vi "Bulk Add Dialog.vi"(8 "error in (no error)":errorcluster, 11 "Type":T1=enum."Input Register") -> (0 "error out":errorcluster, 1 "Cancelled?":bool, 2 "Quantity Out":u16, 3 "Root Name Out":string, 4 "DataType Out":T3, 5 "Starting Address Out":u16, 7 "Pack Values? Out":bool)   [LabVIEW 2020, in "Modbus Master System Explorer.lvlib"]
uses:
  Modbus Master System Explorer.lvlib
  Shared/Controls/Data Model/DataType.ctl
  Radix.ctl
  Modbus Type.ctl
  Shared/Modbus Master Shared.lvlib
panel:
  in  "Radix":T2=enum."Hexidecimal"
  in  "Pack Values?":bool
  in  "DataType":T3=enum."U16"
  in  "Cancel Button":bool
  in  "OK Button":bool
  in  "Quantity":u16
  in  "Starting Address":u16 format="%.0x"
  in  "Root Name":string="Holding Register"
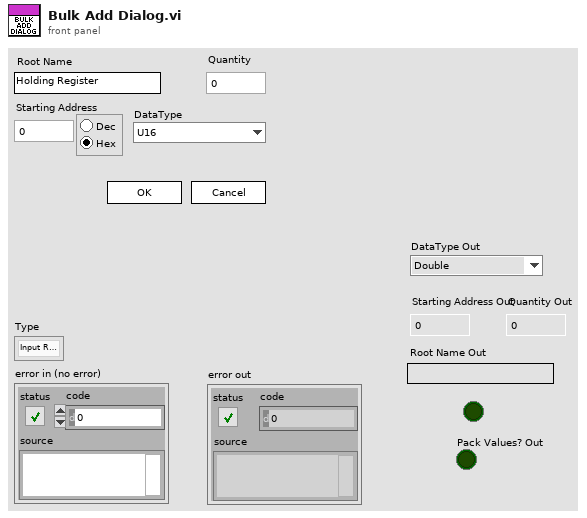
[diagram p1: front panel]
types:
  T1 = typedef "Modbus Master Shared.lvlib/Modbus Type.ctl" = enum16{"Coil", "Discrete Input", "Holding Register", "Input Register"}
  T2 = typedef "Modbus Master System Explorer.lvlib/Radix.ctl" = enum32{"Decimal", "Hexidecimal"}
  T3 = typedef "Modbus Master Shared.lvlib/DataType.ctl" = enum16{"Double", "Single", "I64", "I32", "I16", "I8", "U64", "U32", "U16", "U8", "Boolean"}
  T4 = enum32{"Invalid", "Standard", "Closed", "Hidden", "Minimized", "Maximized"}
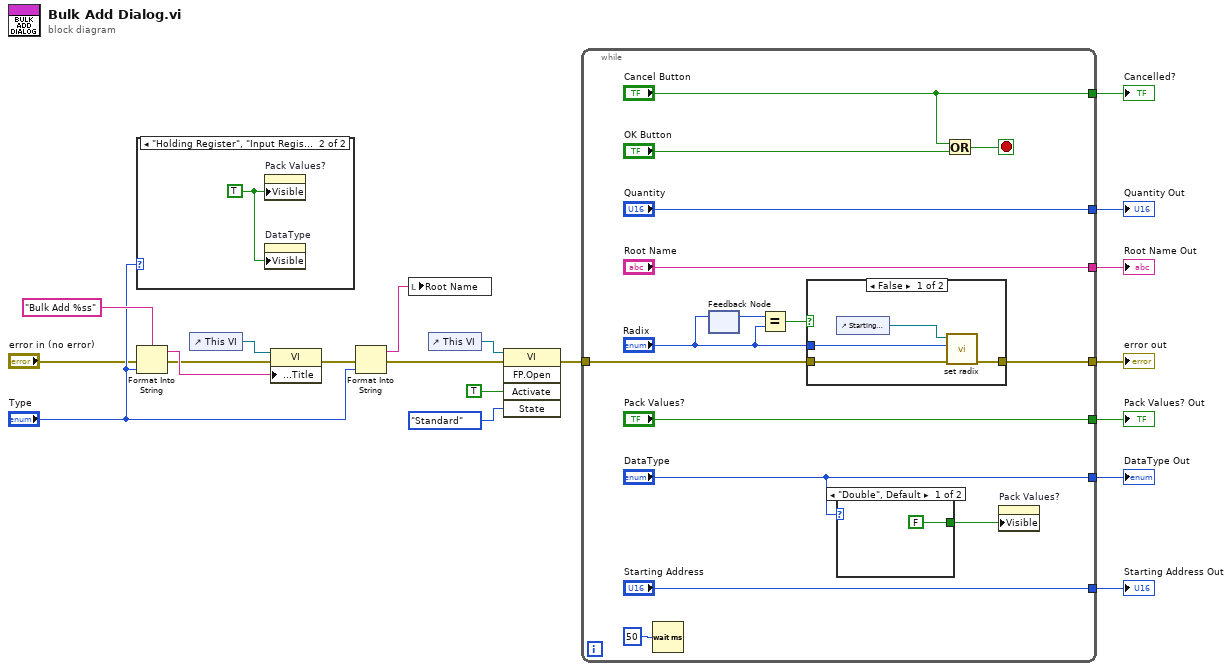
[diagram p0: block diagram]
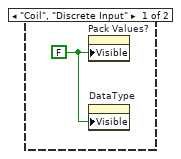
[diagram p2: hidden frame]
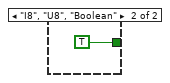
[diagram p4: hidden frame]
diagram:
  n1 = case shown="\"Holding Register\", \"Input Register\"" "Type" {
    frame "Coil", "Discrete Input" {
      w21 = FALSE ("Visible")
      n2 = property on="Pack Values?" class="Bool (strict)"("Visible"=w21) -> ()  [unwired: 2 in, 2 out]
      n3 = property on="DataType" class="Enum (strict)"("Visible"=w21) -> ()  [unwired: 2 in, 2 out]
    }
    frame "Holding Register", "Input Register" {
      w22 = TRUE ("Visible")
      n4 = property on="Pack Values?" class="Bool (strict)"("Visible"=w22) -> ()  [unwired: 2 in, 2 out]
      n5 = property on="DataType" class="Enum (strict)"("Visible"=w22) -> ()  [unwired: 2 in, 2 out]
    }
  }
  n6 = Format Into String(format string="Bulk Add %ss", error in="error in (no error)", "Type") -> (resulting string=w6:string, error out=w2:errorcluster)  [unwired: 1 in]
  n7 = control-ref of="This VI"() -> (w8:refnum<vi>)
  n8 = property class="VI"(reference=w8, error in=w2, "Front Panel.Title"=w6) -> (error out=w3:errorcluster)  [unwired: 1 out]
  n9 = Format Into String(error in=w3, "Type") -> (resulting string=w9:string, error out=w4:errorcluster)  [unwired: 2 in]
  n10 = local write "Root Name"(w9) -> ()
  n11 = control-ref of="This VI"() -> (w16:refnum<vi>)
  n12 = invoke class="VI" method="FP.Open"(reference=w16, error in=w4, "Activate"=TRUE ("Activate?"), "State"=T4."Standard") -> (error out=w13:errorcluster)  [unwired: 1 in, 4 out]
  n13 = while {
    tunnel: ["Cancel Button"] -> w20
    tunnel: ["Root Name"] -> w19
    tunnel: ["Quantity"] -> w18
    tunnel: ["Starting Address"] -> w17
    tunnel: w13 -> [w27]
    tunnel: [w26] -> w12
    tunnel: ["DataType"] -> w11
    tunnel: ["Pack Values?"] -> w10
    stop <- w36 stop-if-true
    n14 = Wait (ms)(milliseconds to wait=u32 50) -> ()  [unwired: 1 out]
    n15 = feedback-in #1("Radix") -> ()
    n16 = feedback #1() -> (w25:T2)  [unwired: 1 in]
    n17 = Equal?(x=w25, y="Radix") -> (x = y?=w23:bool)
    n18 = case shown="False" w23 {
      tunnel: w27 -> [w40 w42]
      tunnel: [w39 w42] -> w26
      tunnel: "Radix" -> [w38 _]
      frame False {
        n19 = control-ref of="Starting Address"() -> (w41:refnum<vi>)
        n20 = call "set radix.vi"("error in (no error)"=w40, "Radix"=w38, "Digital in"=w41) -> ("error out"=w39:errorcluster)  [unwired: 8 in]
      }
      frame True {
      }
    }
    n21 = case shown="\"Double\", Default" "DataType" {
      tunnel: [FALSE ("Visible") TRUE ("Visible")] -> w28
      frame "Double", Default {
      }
      frame "I8", "U8", "Boolean" {
      }
    }
    n22 = Or(x="Cancel Button", y="OK Button") -> (x .or. y?=w36:bool)
    n23 = property on="Pack Values?" class="Bool (strict)"("Visible"=w28) -> ()  [unwired: 2 in, 2 out]
  }
  "error out" <- w12
  "Root Name Out" <- w19
  "Starting Address Out" <- w17
  "Cancelled?" <- w20
  "Quantity Out" <- w18
  "DataType Out" <- w11
  "Pack Values? Out" <- w10
